vi "Find Event Structure from Case Structure.vi"(8 "error in (no error)":errorcluster, 11 "CaseStructure":refnum<vi>) -> (0 "error out":errorcluster, 1 "EvntStruct Refnum":refnum<vi>)   [LabVIEW 2017, in "CSM-Helper Utility.lvlib"]
uses:
  CSM-Helper Utility.lvlib
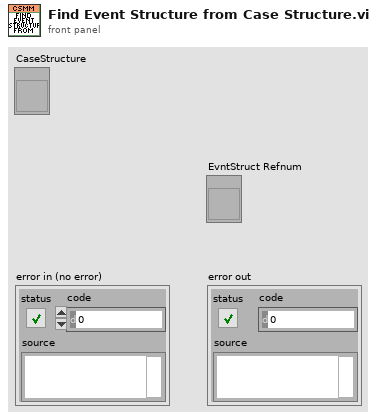
[diagram p1: front panel]
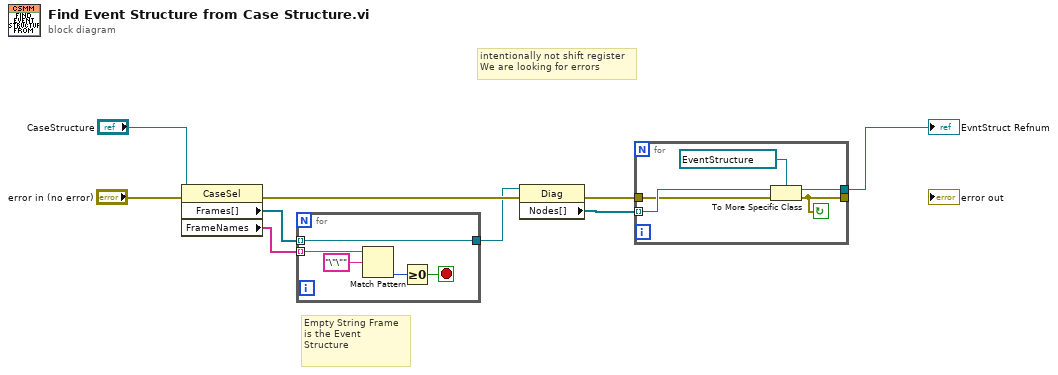
[diagram p0: block diagram]
diagram:
  # "Empty String Frame is the Event Structure"
  # "intentionally not shift register\nWe are looking for errors"
  n1 = property on="Property Node" class="CaseSel"(reference="CaseStructure", error in="error in (no error)") -> (error out=w6:errorcluster, "Frames[]"=w2:refnum<vi>[], "FrameNames"=w3:string[])  [unwired: 1 out]
  n2 = for {
    tunnel: w3 -> [w14] mode=indexing
    tunnel: w2 -> [w10] mode=indexing
    tunnel: [w10] -> w1
    stop <- w11 stop-if-true
    n3 = Match Pattern(string=w14, regular expression="\"\"") -> (offset past match=w12:i32)  [unwired: 1 in, 3 out]
    n4 = Greater Or Equal To 0?(x=w12) -> (x >= 0?=w11:bool)
  }
  n5 = property on="Property Node" class="Diag"(reference=w1, error in=w6) -> (error out=w4:errorcluster, "Nodes[]"=w7:refnum<vi>[])  [unwired: 1 out]
  n6 = for {
    tunnel: w7 -> [w18] mode=indexing
    tunnel: [w17] -> w5
    tunnel: w4 -> [w16]
    tunnel: [w15] -> _
    stop <- w15 continue-if-true
    n7 = To More Specific Class(target class=refnum<vi> refnum ("EvntStruct Refnum"), reference=w18, error in=w16) -> (specific class reference=w17:refnum<vi>, error out=w15:errorcluster)
  }
  "EvntStruct Refnum" <- w5
